vi "getTriggerIn.vi"(8 "error in (no error)":errorcluster, 11 "CCD in":refnum<class "CCD.lvclass">) -> (0 "error out":errorcluster, 1 "signalType":T1=-1 items=["Input Trigger Disabled"=-1, "TTL Falling Edge"=0, "TTL Rising Edge"=1], 2 "event":T2=-1 items=["Input Trigger Disabled"=-1, "Once - Start All"=0, "Each - For Each Acq"=1], 3 "CCD out":refnum<class "CCD.lvclass">, 5 "address":T3=-1 items=["Input Trigger Disabled"=-1, "Trigger Input"=0])   [LabVIEW 2023, in "CCD.lvclass"]
uses:
  CCD.lvclass
  TriggerInAddressRing.ctl
  TriggerInEventRing.ctl
  TriggerInSignalTypeRing.ctl
  TriggerIn.ctl
  20f7d3bd-08ac-4524-9bed-df36c1da25a0.vi
  a21955fc-e3a0-4e36-8495-41f1bfac7860.vi
  <vilib>/JDP Science/JSONtext/Variant to JSON Text.vi
  <vilib>/JDP Science/JSONtext/Set Item.vi
  <vilib>/JDP Science/JSONtext/JSON text to Variant.vi
  <vilib>/JDP Science/JSONtext/LVClass Serializer/JSONtext LVClass Serializer.lvclass
  GenericDevice/GenericDevice.lvclass
panel:
  # "Connector Pane"
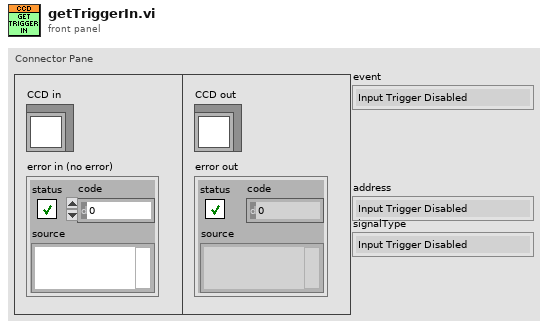
[diagram p1: front panel]
types:
  T1 = typedef "CCD.lvclass/TriggerInSignalTypeRing.ctl" = i32
  T2 = typedef "CCD.lvclass/TriggerInEventRing.ctl" = i32
  T3 = typedef "CCD.lvclass/TriggerInAddressRing.ctl" = i32
  T4 = typedef "CCD.lvclass/TriggerIn.ctl" = cluster{"address":i32, "event":i32, "signalType":i32}
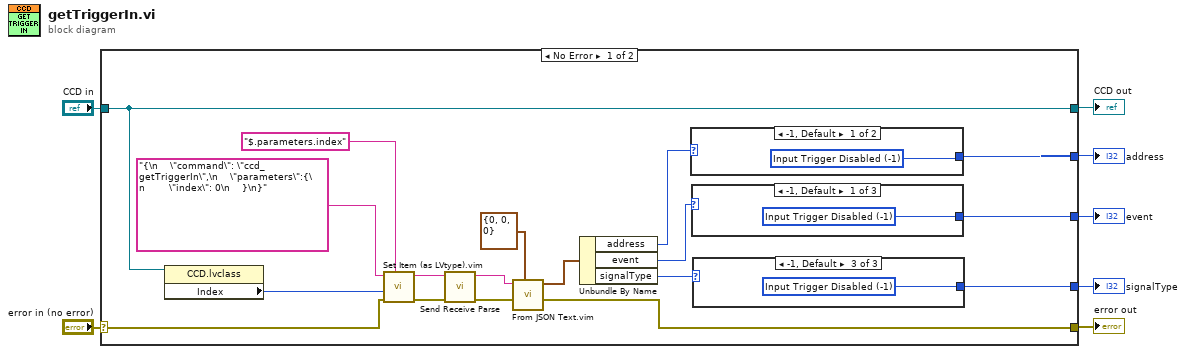
[diagram p0: block diagram]
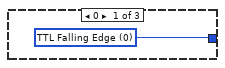
[diagram p2: hidden frame]
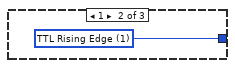
[diagram p3: hidden frame]
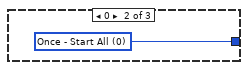
[diagram p4: hidden frame]
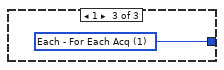
[diagram p5: hidden frame]
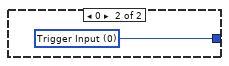
[diagram p6: hidden frame]
diagram:
  n1 = case shown="No Error" "error in (no error)" {
    selector: "error in (no error)" -> [w21 w35]
    tunnel: [w20 w35] -> w6
    tunnel: [w23 w34] -> w4
    tunnel: "CCD in" -> [w23 w34]
    tunnel: [w12 _] -> w3
    tunnel: [w10 _] -> w2
    tunnel: [w8 _] -> w1
    frame No Error {
      n2 = property class="CCD.lvclass"(reference=w23) -> ("Index"=w22:i32)  [unwired: 1 in, 2 out]
      n3 = call "Set Item (as LVtype).vim"("$Path or Item Name"="$.parameters.index", "error in (no error)"=w21, "Anything"=w22, "JSON"="{\n    \"command\": \"ccd_getTriggerIn\",\n    \"parameters\":{\n        \"index\": 0\n    }\n}") -> ("error out"=w17:errorcluster, "<JSON>"=w19:string)  [unwired: 4 in, 1 out]
      n4 = call "Send Receive Parse.vi"("error in"=w17, "<JSON>"=w19) -> ("error out"=w16:errorcluster, "results-JSON string"=w18:string)  [unwired: 7 in, 1 out]
      n5 = call "From JSON Text.vim"("Data Type and Default Value"=T4 {"address"=0, "event"=0, "signalType"=0} ("Trigger Parameters"), "error in (no error)"=w16, "JSON"=w18) -> ("error out"=w20:errorcluster, "Data out"=w14:T4)  [unwired: 7 in]
      n6 = Unbundle By Name(w14) -> ("address"=w13:i32, "event"=w11:i32, "signalType"=w9:i32)
      n7 = case shown="-1, Default" w13 {
        tunnel: [w32 w33] -> w12
        frame -1, Default {
          w32 = T3 -1 items=["Input Trigger Disabled"=-1, "Trigger Input"=0] ("address")
        }
        frame 0 {
          w33 = T3 0 items=["Input Trigger Disabled"=-1, "Trigger Input"=0] ("address")
        }
      }
      n8 = case shown="-1, Default" w11 {
        tunnel: [w29 w30 w31] -> w10
        frame -1, Default {
          w29 = T2 -1 items=["Input Trigger Disabled"=-1, "Once - Start All"=0, "Each - For Each Acq"=1] ("event")
        }
        frame 0 {
          w30 = T2 0 items=["Input Trigger Disabled"=-1, "Once - Start All"=0, "Each - For Each Acq"=1] ("event")
        }
        frame 1 {
          w31 = T2 1 items=["Input Trigger Disabled"=-1, "Once - Start All"=0, "Each - For Each Acq"=1] ("event")
        }
      }
      n9 = case shown="-1, Default" w9 {
        tunnel: [w26 w27 w28] -> w8
        frame 0 {
          w26 = T1 0 items=["Input Trigger Disabled"=-1, "TTL Falling Edge"=0, "TTL Rising Edge"=1] ("signalType")
        }
        frame 1 {
          w27 = T1 1 items=["Input Trigger Disabled"=-1, "TTL Falling Edge"=0, "TTL Rising Edge"=1] ("signalType")
        }
        frame -1, Default {
          w28 = T1 -1 items=["Input Trigger Disabled"=-1, "TTL Falling Edge"=0, "TTL Rising Edge"=1] ("signalType")
        }
      }
    }
    frame Error {
    }
  }
  "error out" <- w6
  "CCD out" <- w4
  "address" <- w3
  "event" <- w2
  "signalType" <- w1
